vi "AdjustDesiredHeading.vi"(8 "Force direction?":bool, 9 "CCW?":bool, 10 "BoatDirection":dbl, 11 "DesiredHeading":dbl) -> (3 "DesiredHeading Altered":dbl)   [LabVIEW 2013]
doc: "In at least one case, the boat needs to turn towards the desired heading \"the long way\". This is when the boat is going too slowly to tack, and should jibe around to the desired heading.\n\nThis VI checks the desired heading and boat heading against the desired direction of turn (CW vs. CCW). If the boat is supposed to turn CW but it is closer to the desired heading going CCW (or vice versa), this VI will output a makeshift Desired Heading that will force the correct turn addition.\n\nThis is necessary because the PID loop around the rudder will point the rudder at the desired heading in the shortest way possible.\n\nEric Schneider, August 2014"
uses:
  Utilities/Math/Angles/Angle/Angle.lvclass
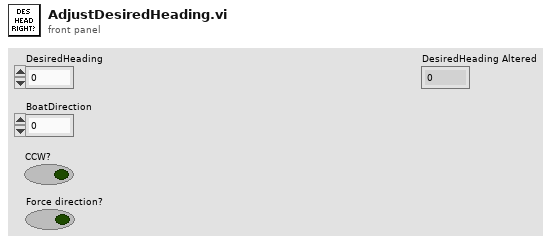
[diagram p1: front panel]
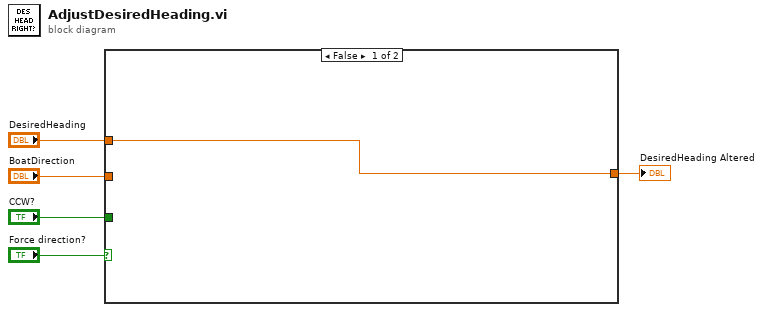
[diagram p0: block diagram]
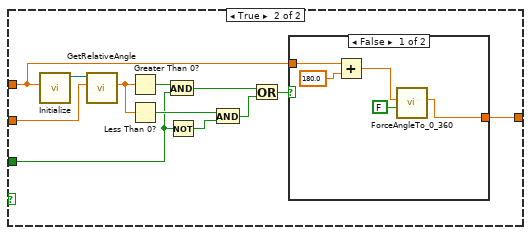
[diagram p2: hidden frame]
diagram:
  n1 = case shown="False" "Force direction?" {
    tunnel: "BoatDirection" -> [_ w17]
    tunnel: "CCW?" -> [_ w12]
    tunnel: "DesiredHeading" -> [w6 w9]
    tunnel: [w6 w8] -> w2
    frame False {
    }
    frame True {
      n2 = call "Initialize.vi"("Input Angle (Deg.)"=w9) -> ("Angle out"=w18:refnum<class "Angle.lvclass">)  [unwired: 9 in, 1 out]
      n3 = call "GetRelativeAngle.vi"("Boat Heading (Deg.)"=w17, "Angle in"=w18) -> ("Relative Angle FROM P2 TO P1 (deg)"=w14:dbl)  [unwired: 6 in, 3 out]
      n4 = Greater Than 0?(x=w14) -> (x > 0?=w16:bool)
      n5 = Less Than 0?(x=w14) -> (x < 0?=w13:bool)
      n6 = And(x=w16, y=w12) -> (x .and. y?=w15:bool)
      n7 = Not(x=w12) -> (.not. x?=w11:bool)
      n8 = And(x=w13, y=w11) -> (x .and. y?=w10:bool)
      n9 = Or(x=w15, y=w10) -> (x .or. y?=w7:bool)
      n10 = case shown="False" w7 {
        tunnel: w9 -> [w23 w24]
        tunnel: [w19 w24] -> w8
        frame False {
          n11 = Add(x=w23, y=180.0) -> (x+y=w21:dbl)
          n12 = call "ForceAngleTo_0_360.vi"("Use angle class? (T)"=FALSE ("Use angle class?"), "Angle in"=w21) -> ("Forced Angle"=w19:dbl)  [unwired: 7 in, 2 out]
        }
        frame True {
          # "If the desired heading is CCW of the boat direction (the relative angle is greater than 0) AND the boat is supposed to be turning CCW then leave the desired heading unaltered. Same with relative angle less than 0 and CW."
        }
      }
    }
  }
  "DesiredHeading Altered" <- w2
